vi "Near Field Motors.vi"() -> ()   [LabVIEW 2014]
doc: "Use this template to build a producer/consumer design pattern with events to produce queue items. Use this design pattern instead of the User Interface Event Handler pattern for user interfaces when you want to execute code asynchronously in response to an event without slowing the user interface responsiveness."
panel:
  out "File error out":errorcluster
  in  "RefLabels 4":string(combo) caption="M4"
  in  "RefLabels 3":string(combo) caption="M3"
  in  "RefLabels 2":string(combo) caption="M2"
  in  "All refs":dbl[][](array[numeric]) format="%.6f"
  in  "RefLabels 1":string(combo) caption="M1"
  in  "Referencing mode":T1(array[ring])=[enum."FRF (-> FNL)", enum."FRF (-> FNL)", enum."FRF (-> FNL)", enum."FRF (-> FNL)"]
  out "Host address":string
  out "Message":string
  out "Identification":string
  out "PI error out":errorcluster
  in  "Save References":bool
  in  "Set 4":bool caption="Set4"
  in  "Go 4":bool caption="Go4"
  in  "Set 3":bool caption="Set3"
  in  "Go 3":bool caption="Go3"
  in  "Set 2":bool caption="Set2"
  in  "Go 2":bool caption="Go2"
  in  "Go 1":bool caption="Go1"
  in  "Set 1":bool caption="Set1"
  in  "Ref Values":dbl[](array[numeric]) format="%.6f"
  in  "Max Pos":dbl[](array[numeric]) format="%.6f"
  in  "Min Pos":dbl[](array[numeric]) format="%.6f"
  in  "MOVE":bool
  in  "stop motors":bool
  out "Current position":dbl[](array[numeric]) format="%.6f"
  in  "Absolute \ntarget position":dbl[](array[numeric]) format="%.6f"
  in  "MV -":bool
  in  "Relative distance to mv":dbl format="%#_g mm"
  in  "Axis to move":T2(ring)
  in  "MV+":bool
  out "Init OK":bool
  in  "Axes to move":string[](array[string])
  out "+/- movement\nrange":dbl[](array[numeric]) format="%.6f"
  out "Referencing\nin progress":bool
  out "Conn. \nAxes":string[](array[string])
  in  "All Axes?":bool=TRUE
  in  "Stage selection":T3={"Force?"=FALSE, "Dialog?"=TRUE, "Stages"=[]}
  out "Position":dbl[](array[numeric]) format="%.6f"
  out "Referencing\nsuccessful?":bool[](array[boolean])
  in  "Reference Motors":bool
  in  "stop":bool
  # "M1: Horizontal NF"
  # "M2: Vertical NF"
  # "<unassigned>"
  # "<unassigned>"
  # "M1: Horizontal NF"
  # "M2: Vertical NF"
  # "<unassigned>"
  # "<unassigned>"
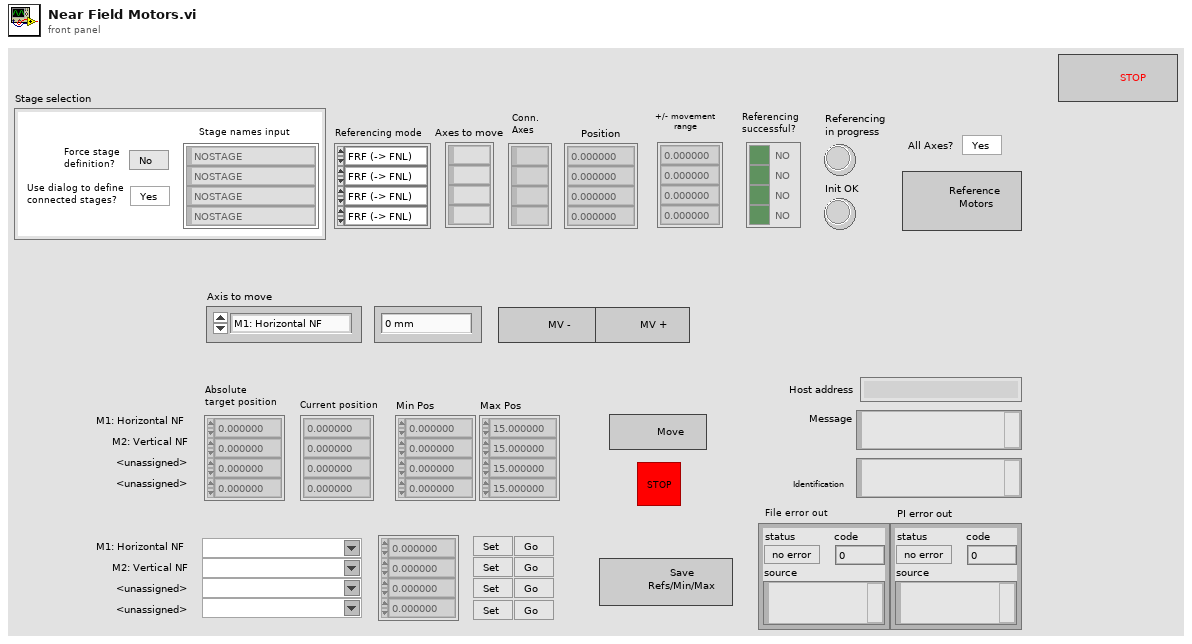
[diagram p1: front panel]
types:
  T1 = enum16{"FRF (-> FNL)", "FRF", "FNL", "FPL", "RON OFF"}[]
  T2 = enum16{"M1: Horizontal NF", "M2 : Vertical NF", "M3 : <unassigned> ", "M4 : <unassigned>"}
  T3 = cluster{"Force?":bool, "Dialog?":bool, "Stages":string[]}
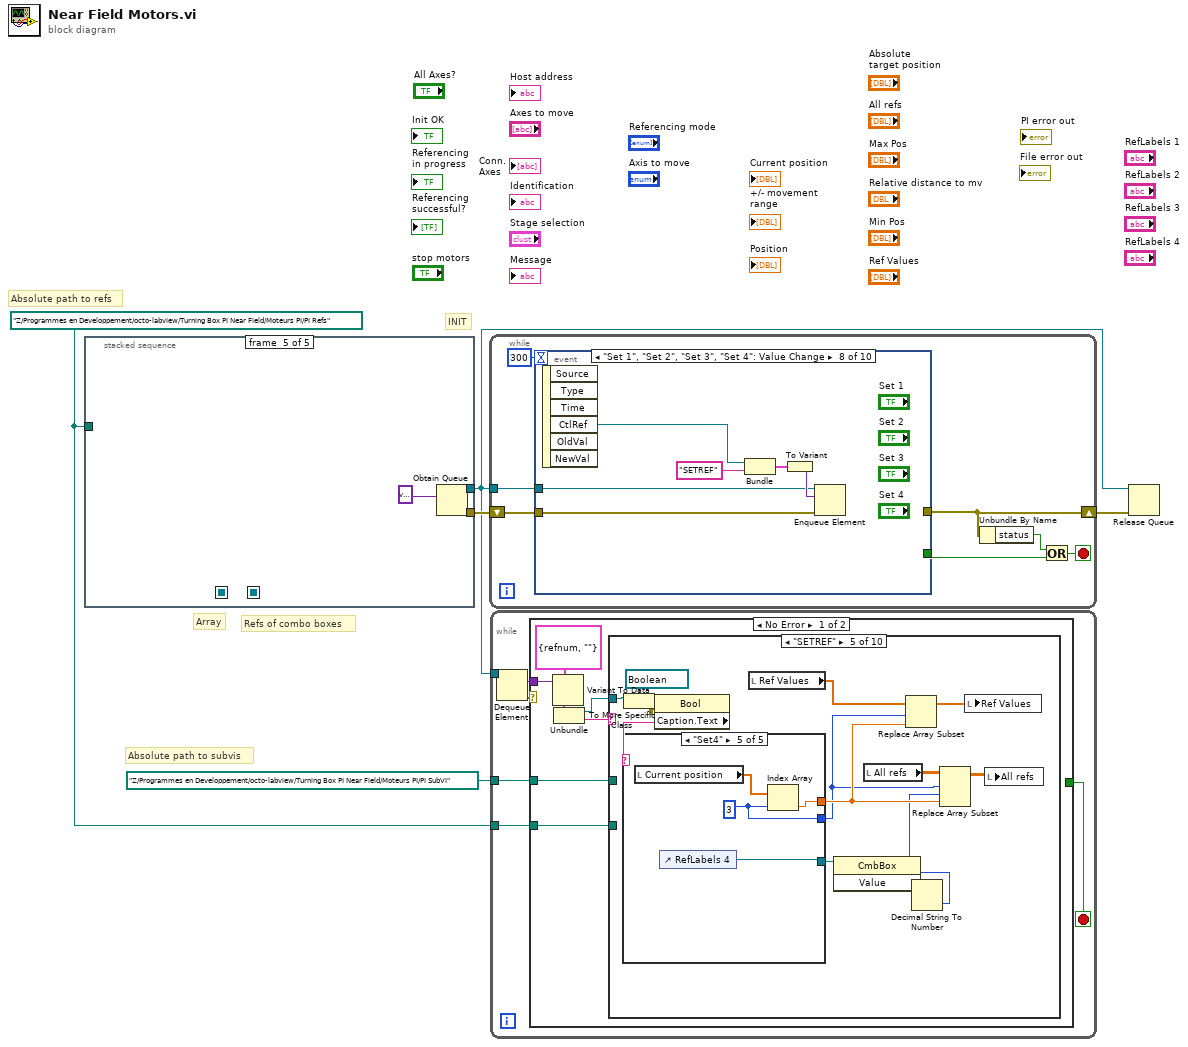
[diagram p0: block diagram]
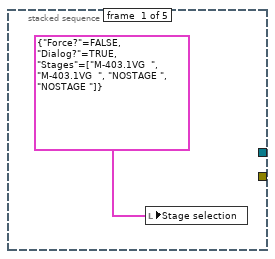
[diagram p2: hidden frame]
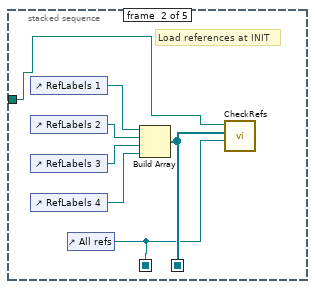
[diagram p3: hidden frame]
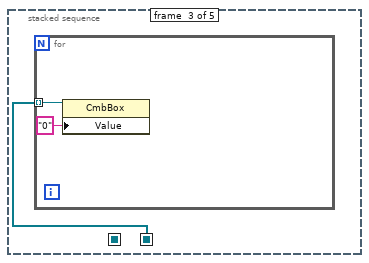
[diagram p4: hidden frame]
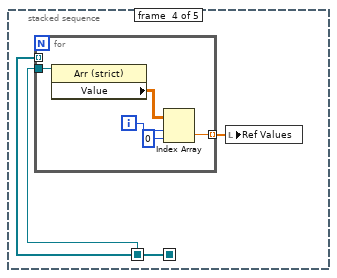
[diagram p5: hidden frame]
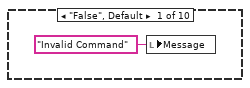
[diagram p6: hidden frame]
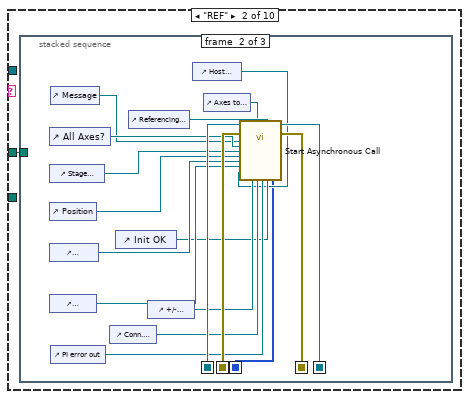
[diagram p7: hidden frame]
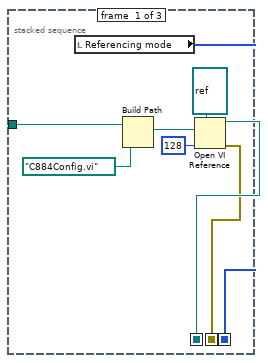
[diagram p8: hidden frame]
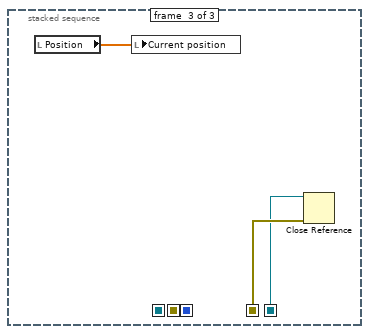
[diagram p9: hidden frame]
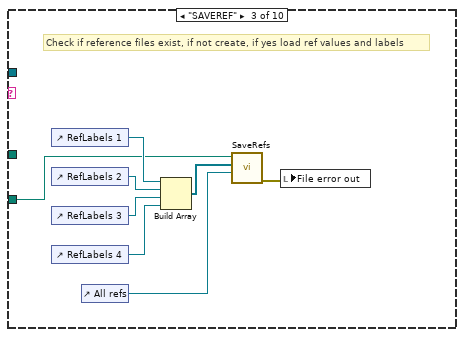
[diagram p10: hidden frame]
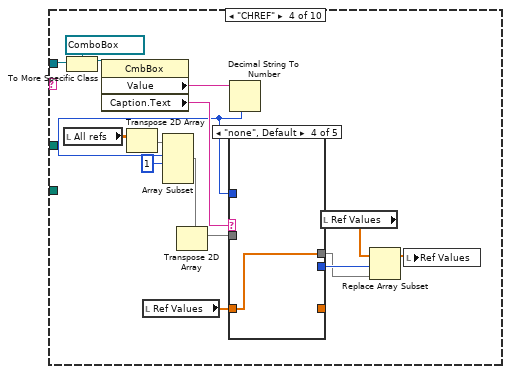
[diagram p11: hidden frame]
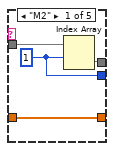
[diagram p12: hidden frame]
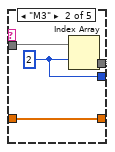
[diagram p13: hidden frame]
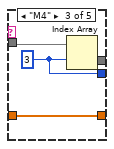
[diagram p14: hidden frame]
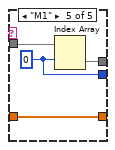
[diagram p15: hidden frame]
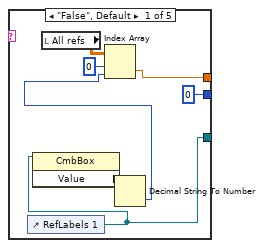
[diagram p16: hidden frame]
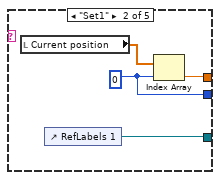
[diagram p17: hidden frame]
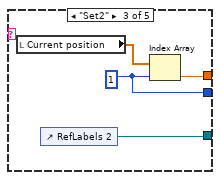
[diagram p18: hidden frame]
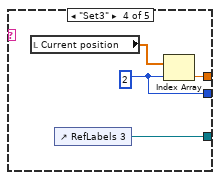
[diagram p19: hidden frame]
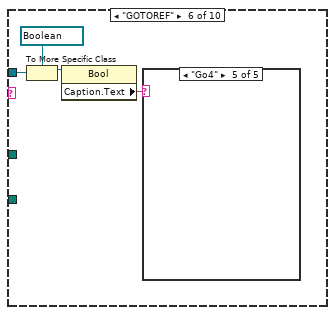
[diagram p20: hidden frame]
diagram:
  w1 = path "Z:/Programmes en Developpement/octo-labview/Turning Box PI Near Field/Moteurs PI/PI Refs" ("vi path")
  # "Refs of combo boxes"
  # "Array"
  # "Absolute path to refs"
  # "Absolute path to subvis"
  # "INIT"
  n1 = stacked-sequence {
    seq-local: [_ w8 _ _ _] -> [_ _ w14 w19 _]
    seq-local: [_ w7 _ _ _] -> [_ _ _ w18 _]
    tunnel: [_ _ _ _ w27] -> w5
    tunnel: [_ _ _ _ w26] -> w3
    tunnel: w1 -> [_ w9 _ _ _]
    frame #0 {
      n2 = local write "Stage selection"(T3 {"Force?"=FALSE, "Dialog?"=TRUE, "Stages"=["M-403.1VG  ", "M-403.1VG  ", "NOSTAGE ", "NOSTAGE "]} ("Stage selection")) -> ()
    }
    frame #1 {
      # "Load references at INIT"
      n3 = control-ref of="RefLabels 1"() -> (w10:refnum<vi>)
      n4 = control-ref of="RefLabels 2"() -> (w11:refnum<vi>)
      n5 = control-ref of="RefLabels 3"() -> (w12:refnum<vi>)
      n6 = control-ref of="RefLabels 4"() -> (w13:refnum<vi>)
      n7 = control-ref of="All refs"() -> (w7:refnum<vi>)
      n8 = Build Array(w10, w11, w12, w13) -> (w8:refnum<vi>[])
      n9 = call "CheckRefs.vi"("All Refs Array Refnum"=w7, "Array of label refnums"=w8, "Path to refs"=w9) -> ()  [unwired: 8 in, 1 out]
    }
    frame #2 {
      n10 = for {
        tunnel: w14 -> [w16] mode=indexing
        n11 = property class="CmbBox"(reference=w16, "Value"="0") -> ()  [unwired: 1 in, 2 out]
      }
    }
    frame #3 {
      n12 = for {
        tunnel: w19 -> [_] mode=indexing
        tunnel: w18 -> [w24]
        tunnel: [w20] -> w17 mode=indexing
        i -> [w22]
        n13 = property class="Arr (strict)"(reference=w24) -> ("Value"=w23:dbl[][])  [unwired: 1 in, 2 out]
        n14 = Index Array(array=w23, index (row)=w22, index (col)=0 ("disabled index (col)")) -> (element=w20:dbl)
      }
      n15 = local write "Ref Values"(w17) -> ()
    }
    frame #4 {
      n16 = Obtain Queue(element data type=variant) -> (queue out=w26:refnum<queue>, error out=w27:errorcluster)  [unwired: 4 in, 1 out]
    }
  }
  n17 = while {
    shift-right: [w30] -> w4
    shift-left: w5 -> [w33]
    tunnel: w3 -> [w34]
    stop <- w31 stop-if-true
    n18 = event shown="[7] \"Set 1\", \"Set 2\", \"Set 3\", \"Set 4\": Value Change" {
      selector: _ -> [_ _ _ _ _ _ _ _ _ _]
      dyn-events: _ -> [_ _ _ _ _ _ _ _ _ _]
      timeout: 300 -> [_ _ _ _ _ _ _ _ _ _]
      tunnel: w34 -> [w40 w46 w52 w58 w64 w69 w75 w78 w84 _]
      tunnel: w33 -> [w39 w45 w51 w57 w63 w70 w74 w77 w83 w89]
      tunnel: [_ _ _ _ _ _ _ _ _ w89] -> w30
      tunnel: [_ _ _ _ _ _ _ _ _ "stop"] -> w32
      event "Reference Motors": Value Change {
        n19 = event-data() -> ()  [unwired: 1 in, 1 out]
        n20 = Bundle("CtlRef"=refnum<vi> refnum, "element"="REF") -> (w36:cluster{"CtlRef":refnum<vi>, "element":string})  [unwired: 1 in]
        n21 = To Variant(anything=w36) -> (Variant=w38:variant)
        n22 = Enqueue Element(queue=w40, element=w38, error in (no error)=w39) -> ()  [unwired: 1 in, 3 out]
      }
      event Timeout {
        n23 = event-data() -> ()  [unwired: 1 in, 1 out]
        n24 = Bundle("CtlRef"=refnum<vi> refnum, "element"="POS?") -> (w42:cluster{"CtlRef":refnum<vi>, "element":string})  [unwired: 1 in]
        n25 = To Variant(anything=w42) -> (Variant=w44:variant)
        n26 = Enqueue Element(queue=w46, element=w44, error in (no error)=w45) -> ()  [unwired: 1 in, 3 out]
      }
      event "MV+": Value Change {
        n27 = event-data() -> ()  [unwired: 1 in, 1 out]
        n28 = Bundle("CtlRef"=refnum<vi> refnum, "element"="MVR +") -> (w48:cluster{"CtlRef":refnum<vi>, "element":string})  [unwired: 1 in]
        n29 = To Variant(anything=w48) -> (Variant=w50:variant)
        n30 = Enqueue Element(queue=w52, element=w50, error in (no error)=w51) -> ()  [unwired: 1 in, 3 out]
      }
      event "MV -": Value Change {
        n31 = event-data() -> ()  [unwired: 1 in, 2 out]
        n32 = Bundle("CtlRef"=refnum<vi> refnum, "element"="MVR -") -> (w54:cluster{"CtlRef":refnum<vi>, "element":string})  [unwired: 1 in]
        n33 = To Variant(anything=w54) -> (Variant=w56:variant)
        n34 = Enqueue Element(queue=w58, element=w56, error in (no error)=w57) -> ()  [unwired: 1 in, 3 out]
      }
      event "MOVE": Value Change {
        n35 = event-data() -> ()  [unwired: 1 in, 2 out]
        n36 = Bundle("CtlRef"=refnum<vi> refnum, "element"="MVABS") -> (w60:cluster{"CtlRef":refnum<vi>, "element":string})  [unwired: 1 in]
        n37 = To Variant(anything=w60) -> (Variant=w62:variant)
        n38 = Enqueue Element(queue=w64, element=w62, error in (no error)=w63) -> ()  [unwired: 1 in, 3 out]
      }
      event "Save References": Value Change {
        n39 = event-data() -> ()  [unwired: 1 in, 2 out]
        n40 = Bundle("CtlRef"=refnum<vi> refnum, "element"="SAVEREF") -> (w66:cluster{"CtlRef":refnum<vi>, "element":string})  [unwired: 1 in]
        n41 = To Variant(anything=w66) -> (Variant=w68:variant)
        n42 = Enqueue Element(queue=w69, element=w68, error in (no error)=w70) -> ()  [unwired: 1 in, 3 out]
      }
      event "RefLabels 1", "RefLabels 2", "RefLabels 3", "RefLabels 4": Value Change {
        n43 = event-data() -> ("CtlRef"=w71:refnum<vi>)  [unwired: 1 in, 5 out]
        n44 = Bundle("CtlRef"=w71, "element"="CHREF") -> (w73:cluster{"CtlRef":refnum<vi>, "element":string})  [unwired: 1 in]
        n45 = To Variant(anything=w73) -> (Variant=w72:variant)
        n46 = Enqueue Element(queue=w75, element=w72, error in (no error)=w74) -> ()  [unwired: 1 in, 3 out]
      }
      event "Set 1", "Set 2", "Set 3", "Set 4": Value Change {
        n47 = event-data() -> ("CtlRef"=w79:refnum<vi>)  [unwired: 1 in, 5 out]
        n48 = Bundle("CtlRef"=w79, "element"="SETREF") -> (w81:cluster{"CtlRef":refnum<vi>, "element":string})  [unwired: 1 in]
        n49 = To Variant(anything=w81) -> (Variant=w80:variant)
        n50 = Enqueue Element(queue=w78, element=w80, error in (no error)=w77) -> ()  [unwired: 1 in, 3 out]
      }
      event "Go 1", "Go 2", "Go 3", "Go 4": Value Change {
        n51 = event-data() -> ("CtlRef"=w85:refnum<vi>)  [unwired: 1 in, 5 out]
        n52 = Bundle("CtlRef"=w85, "element"="GOTOREF") -> (w87:cluster{"CtlRef":refnum<vi>, "element":string})  [unwired: 1 in]
        n53 = To Variant(anything=w87) -> (Variant=w86:variant)
        n54 = Enqueue Element(queue=w84, element=w86, error in (no error)=w83) -> ()  [unwired: 1 in, 3 out]
      }
      event "stop": Value Change {
        n55 = event-data() -> ()  [unwired: 1 in, 1 out]
      }
    }
    n56 = Unbundle By Name(w30) -> ("status"=w29:bool)
    n57 = Or(x=w29, y=w32) -> (x .or. y?=w31:bool)
  }
  n58 = while {
    tunnel: w3 -> [w96]
    tunnel: path "Z:/Programmes en Developpement/octo-labview/Turning Box PI Near Field/Moteurs PI/PI SubVI" ("vi path") -> [w92]
    tunnel: w1 -> [w91]
    stop <- w93 stop-if-true
    n59 = Dequeue Element(queue=w96) -> (element=w94:variant, error out=w95:errorcluster)  [unwired: 2 in, 2 out]
    n60 = case shown="No Error" w95 {
      tunnel: w94 -> [w101 _]
      tunnel: [_ TRUE] -> w93
      tunnel: w92 -> [w103 _]
      tunnel: w91 -> [w102 _]
      frame No Error {
        n61 = Variant To Data(type=cluster{"CtlRef":refnum<vi>, "element":string} {"CtlRef"=refnum, "element"=""} ("cluster"), Variant=w101) -> (data=w100:cluster{"CtlRef":refnum<vi>, "element":string})  [unwired: 1 in, 1 out]
        n62 = Unbundle(w100) -> ("CtlRef"=w98:refnum<vi>, "element"=w99:string)
        n63 = case shown="\"SETREF\"" w99 {
          tunnel: w103 -> [_ w105 _ _ _ _ w217 w239 w267 _]
          tunnel: w102 -> [_ _ w138 _ _ _ _ _ _ _]
          tunnel: w98 -> [_ _ _ w158 w189 w216 _ _ _ _]
          frame "False", Default {
            n64 = local write "Message"("Invalid Command" ("Message")) -> ()
          }
          frame "REF" {
            n65 = stacked-sequence {
              seq-local: [w111 _ _] -> [_ w131 _]
              seq-local: [w110 _ _] -> [_ w130 _]
              seq-local: [_ w117 _] -> [_ _ w134]
              seq-local: [_ w116 _] -> [_ _ w133]
              seq-local: [w106 _ _] -> [_ w114 _]
              tunnel: w105 -> [w109 _ _]
              frame #0 {
                n66 = local read "Referencing mode"() -> (w106:T1)
                n67 = Build Path(base path=w109, name or relative path=path "C884Config.vi" ("vi path")) -> (appended path=w107:path)
                n68 = Open VI Reference(type specifier VI Refnum (for type only)=refnum<vi> refnum, vi path=w107, options=128) -> (vi reference=w111:refnum<vi>, error out=w110:errorcluster)  [unwired: 3 in]
              }
              frame #1 {
                n69 = control-ref of="All Axes?"() -> (w129:refnum<vi>)
                n70 = control-ref of="Stage selection"() -> (w122:refnum<vi>)
                n71 = control-ref of="Position"() -> (w128:refnum<vi>)
                n72 = control-ref of="Identification"() -> (w127:refnum<vi>)
                n73 = control-ref of="Referencing\nsuccessful?"() -> (w126:refnum<vi>)
                n74 = control-ref of="Message"() -> (w119:refnum<vi>)
                n75 = control-ref of="PI error out"() -> (w123:refnum<vi>)
                n76 = control-ref of="Conn. \nAxes"() -> (w124:refnum<vi>)
                n77 = control-ref of="Init OK"() -> (w118:refnum<vi>)
                n78 = control-ref of="Referencing\nin progress"() -> (w121:refnum<vi>)
                n79 = control-ref of="+/- movement\nrange"() -> (w125:refnum<vi>)
                n80 = control-ref of="Host address"() -> (w115:refnum<vi>)
                n81 = control-ref of="Axes to move"() -> (w120:refnum<vi>)
                n82 = call-by-ref "Start Asynchronous Call"(reference=w131, error in=w130, "All axes? Refnum"=w129, "Stages Selection Refnum"=w122, "Position Refnum"=w128, "Identification Refnum"=w127, "Referencing successful Refnum"=w126, "Host Addresss Refnum"=w115, "Message Out Refnum"=w119, "+/- mvt range Refnum"=w125, "Axes to Move Refnum"=w120, "Connected Axes Refnum"=w124, "Referencing mode"=w114, "Error OUT Refnum"=w123, "En cours LED Refnum"=w121, "LED Initialis. OK? Refnum"=w118) -> (reference out=w116:refnum<vi>, error out=w117:errorcluster)  [unwired: 6 in]
              }
              frame #2 {
                n83 = local read "Position"() -> (w132:dbl[])
                n84 = local write "Current position"(w132) -> ()
                n85 = Close Reference(reference=w133, error in (no error)=w134) -> ()  [unwired: 1 out]
              }
            }
          }
          frame "SAVEREF" {
            # "Check if reference files exist, if not create, if yes load ref values and labels"
            n86 = control-ref of="RefLabels 1"() -> (w142:refnum<vi>)
            n87 = control-ref of="RefLabels 2"() -> (w141:refnum<vi>)
            n88 = control-ref of="RefLabels 3"() -> (w140:refnum<vi>)
            n89 = control-ref of="RefLabels 4"() -> (w139:refnum<vi>)
            n90 = control-ref of="All refs"() -> (w136:refnum<vi>)
            n91 = Build Array(w142, w141, w140, w139) -> (w137:refnum<vi>[])
            n92 = call "SaveRefs.vi"("All Refs Array Refnum"=w136, "Array of label refnums"=w137, "Path to refs"=w138) -> ("error out"=w135:errorcluster)  [unwired: 8 in]
            n93 = local write "File error out"(w135) -> ()
          }
          frame "CHREF" {
            n94 = local read "All refs"() -> (w153:dbl[][])
            n95 = To More Specific Class(target class=refnum<vi> refnum ("CtlRef"), reference=w158) -> (specific class reference=w156:refnum<vi>)  [unwired: 1 in, 1 out]
            n96 = property class="CmbBox"(reference=w156) -> ("Value"=w155:string, "Caption.Text"=w154:string)  [unwired: 1 in, 2 out]
            n97 = Transpose 2D Array(2D array=w153) -> (transposed array=w152:dbl[][])
            n98 = local read "Ref Values"() -> (w147:dbl[])
            n99 = Decimal String To Number(string=w155) -> (number=w151:i32)  [unwired: 2 in, 1 out]
            n100 = Array Subset(array=w152, index (row)=w151, length (row)=1 ("length")) -> (w149:dbl[][])  [unwired: 2 in]
            n101 = Transpose 2D Array(2D array=w149) -> (transposed array=w148:dbl[][])
            n102 = case shown="\"none\", Default" w154 {
              tunnel: w151 -> [_ _ _ _ _]
              tunnel: w148 -> [w162 w166 w170 _ w175]
              tunnel: [w161 w164 w168 _ w174] -> w145
              tunnel: [w160 w165 w169 w171 w173] -> w144
              tunnel: w147 -> [w159 w163 w167 w171 w172]
              tunnel: [w159 w163 w167 _ w172] -> _
              frame "M2" {
                w161 = 1
                n103 = Index Array(array=w162, index (row)=w161) -> (element=w160:dbl[])  [unwired: 1 in]
              }
              frame "M3" {
                w164 = 2
                n104 = Index Array(array=w166, index (row)=w164) -> (element=w165:dbl[])  [unwired: 1 in]
              }
              frame "M4" {
                w168 = 3
                n105 = Index Array(array=w170, index (row)=w168) -> (element=w169:dbl[])  [unwired: 1 in]
              }
              frame "none", Default {
              }
              frame "M1" {
                w174 = 0
                n106 = Index Array(array=w175, index (row)=w174) -> (element=w173:dbl[])  [unwired: 1 in]
              }
            }
            n107 = local read "Ref Values"() -> (w146:dbl[])
            n108 = Replace Array Subset(array=w146, new element=w144, index=w145) -> (w143:dbl[])
            n109 = local write "Ref Values"(w143) -> ()
          }
          frame "SETREF" {
            n110 = To More Specific Class(target class=refnum<vi> refnum ("CtlRef"), reference=w189) -> (specific class reference=w187:refnum<vi>, error out=w186:errorcluster)  [unwired: 1 in]
            n111 = property class="Bool"(reference=w187, error in=w186) -> ("Caption.Text"=w185:string)  [unwired: 2 out]
            n112 = case shown="\"Set4\"" w185 {
              tunnel: [w191 w199 w203 w207 w211] -> w178
              tunnel: [0 w198 w202 w206 w210] -> w176
              tunnel: [w190 w197 w201 w205 w209] -> w179
              frame "False", Default {
                n113 = control-ref of="RefLabels 1"() -> (w190:refnum<vi>)
                n114 = property class="CmbBox"(reference=w190) -> ("Value"=w195:string)  [unwired: 1 in, 2 out]
                n115 = local read "All refs"() -> (w196:dbl[][])
                n116 = Decimal String To Number(string=w195) -> (number=w192:i32)  [unwired: 2 in, 1 out]
                n117 = Index Array(array=w196, index (row)=0, index (col)=w192) -> (element=w191:dbl)
              }
              frame "Set1" {
                w198 = 0
                n118 = local read "Current position"() -> (w200:dbl[])
                n119 = control-ref of="RefLabels 1"() -> (w197:refnum<vi>)
                n120 = Index Array(array=w200, index=w198) -> (element=w199:dbl)
              }
              frame "Set2" {
                w202 = 1
                n121 = local read "Current position"() -> (w204:dbl[])
                n122 = control-ref of="RefLabels 2"() -> (w201:refnum<vi>)
                n123 = Index Array(array=w204, index=w202) -> (element=w203:dbl)
              }
              frame "Set3" {
                w206 = 2
                n124 = local read "Current position"() -> (w208:dbl[])
                n125 = control-ref of="RefLabels 3"() -> (w205:refnum<vi>)
                n126 = Index Array(array=w208, index=w206) -> (element=w207:dbl)
              }
              frame "Set4" {
                w210 = 3
                n127 = local read "Current position"() -> (w212:dbl[])
                n128 = control-ref of="RefLabels 4"() -> (w209:refnum<vi>)
                n129 = Index Array(array=w212, index=w210) -> (element=w211:dbl)
              }
            }
            n130 = local read "Ref Values"() -> (w183:dbl[])
            n131 = property class="CmbBox"(reference=w179) -> ("Value"=w184:string)  [unwired: 1 in, 2 out]
            n132 = local read "All refs"() -> (w182:dbl[][])
            n133 = Replace Array Subset(array=w183, new element=w178, index=w176) -> (w180:dbl[])
            n134 = Decimal String To Number(string=w184) -> (number=w177:i32)  [unwired: 2 in, 1 out]
            n135 = Replace Array Subset(array=w182, new element=w178, index (row)=w176, index (col)=w177) -> (w181:dbl[][])
            n136 = local write "Ref Values"(w180) -> ()
            n137 = local write "All refs"(w181) -> ()
          }
          frame "GOTOREF" {
            n138 = To More Specific Class(target class=refnum<vi> refnum ("CtlRef"), reference=w216) -> (specific class reference=w214:refnum<vi>)  [unwired: 1 in, 1 out]
            n139 = property class="Bool"(reference=w214) -> ("Caption.Text"=w213:string)  [unwired: 1 in, 2 out]
            n140 = case shown="\"Go4\"" w213 {
              frame "False", Default {
              }
              frame "Go1" {
              }
              frame "Go2" {
              }
              frame "Go3" {
              }
              frame "Go4" {
              }
            }
          }
          frame "MVABS" {
            n141 = stacked-sequence {
              seq-local: [w220 _ _] -> [_ w236 _]
              seq-local: [w219 _ _] -> [_ w235 _]
              seq-local: [_ w227 _] -> [_ _ w238]
              seq-local: [_ w226 _] -> [_ _ w237]
              seq-local: [w218 _ _] -> [_ w225 _]
              tunnel: w217 -> [w222 _ _]
              frame #0 {
                n142 = local read "Absolute \ntarget position"() -> (w218:dbl[])
                n143 = Build Path(base path=w222, name or relative path=path "MoveSinglePIMotor_C884.vi" ("vi path")) -> (appended path=w221:path)
                n144 = Open VI Reference(type specifier VI Refnum (for type only)=refnum<vi> refnum, vi path=w221) -> (vi reference=w220:refnum<vi>, error out=w219:errorcluster)  [unwired: 4 in]
              }
              frame #1 {
                n145 = control-ref of="stop motors"() -> (w228:refnum<vi>)
                n146 = call-by-ref "Start Asynchronous Call"(reference=w236, error in=w235, "System no."=1, "Move"=w225, "Define home"=FALSE, "Move relative (-)"=FALSE, "Go home"=FALSE, "Move relative (+)"=FALSE ("Move relative (-)"), "Move absolute"=TRUE ("Move relative (-)"), "Stop refnum"=w228) -> (reference out=w227:refnum<vi>, error out=w226:errorcluster)  [unwired: 10 in, 2 out]
              }
              frame #2 {
                n147 = Close Reference(reference=w238, error in (no error)=w237) -> ()  [unwired: 1 out]
              }
            }
          }
          frame "MVR +" {
            n148 = stacked-sequence {
              seq-local: [w247 _ _] -> [_ w264 _]
              seq-local: [w246 _ _] -> [_ w263 _]
              seq-local: [_ w255 _] -> [_ _ w266]
              seq-local: [_ w254 _] -> [_ _ w265]
              seq-local: [w244 _ _] -> [_ w252 _]
              seq-local: [w240 _ _] -> [_ w253 _]
              tunnel: w239 -> [w249 _ _]
              frame #0 {
                n149 = local read "Axis to move"() -> (w242:T2)
                n150 = local read "Relative distance to mv"() -> (w245:dbl)
                n151 = local read "Conn. \nAxes"() -> (w243:string[])
                n152 = Index Array(array=w243, index=w242) -> (element=w241:string)
                n153 = Build Path(base path=w249, name or relative path=path "MoveSinglePIMotor_C884.vi" ("vi path")) -> (appended path=w248:path)
                n154 = Build Array(w245) -> (w244:dbl[])
                n155 = Build Array(w241) -> (w240:string[])
                n156 = Open VI Reference(type specifier VI Refnum (for type only)=refnum<vi> refnum, vi path=w248) -> (vi reference=w247:refnum<vi>, error out=w246:errorcluster)  [unwired: 4 in]
              }
              frame #1 {
                n157 = control-ref of="stop motors"() -> (w256:refnum<vi>)
                n158 = call-by-ref "Start Asynchronous Call"(reference=w264, error in=w263, "System no."=1, "Axes to move"=w253, "Move"=w252, "Define home"=FALSE, "Move relative (-)"=FALSE, "Go home"=FALSE, "Move relative (+)"=TRUE ("Move relative (-)"), "Move absolute"=FALSE ("Move relative (-)"), "Stop refnum"=w256) -> (reference out=w255:refnum<vi>, error out=w254:errorcluster)  [unwired: 9 in, 2 out]
              }
              frame #2 {
                n159 = Close Reference(reference=w266, error in (no error)=w265) -> ()  [unwired: 1 out]
              }
            }
          }
          frame "MVR -" {
            n160 = stacked-sequence {
              seq-local: [w275 _ _] -> [_ w292 _]
              seq-local: [w274 _ _] -> [_ w291 _]
              seq-local: [_ w283 _] -> [_ _ w294]
              seq-local: [_ w282 _] -> [_ _ w293]
              seq-local: [w272 _ _] -> [_ w280 _]
              seq-local: [w268 _ _] -> [_ w281 _]
              tunnel: w267 -> [w277 _ _]
              frame #0 {
                n161 = local read "Axis to move"() -> (w270:T2)
                n162 = local read "Conn. \nAxes"() -> (w271:string[])
                n163 = local read "Relative distance to mv"() -> (w273:dbl)
                n164 = Index Array(array=w271, index=w270) -> (element=w269:string)
                n165 = Build Path(base path=w277, name or relative path=path "MoveSinglePIMotor_C884.vi" ("vi path")) -> (appended path=w276:path)
                n166 = Build Array(w269) -> (w268:string[])
                n167 = Build Array(w273) -> (w272:dbl[])
                n168 = Open VI Reference(type specifier VI Refnum (for type only)=refnum<vi> refnum, vi path=w276) -> (vi reference=w275:refnum<vi>, error out=w274:errorcluster)  [unwired: 4 in]
              }
              frame #1 {
                n169 = control-ref of="stop motors"() -> (w284:refnum<vi>)
                n170 = call-by-ref "Start Asynchronous Call"(reference=w292, error in=w291, "System no."=1, "Axes to move"=w281, "Move"=w280, "Define home"=FALSE, "Move relative (-)"=TRUE, "Go home"=FALSE, "Move relative (+)"=FALSE ("Move relative (-)"), "Move absolute"=FALSE ("Move relative (-)"), "Stop refnum"=w284) -> (reference out=w283:refnum<vi>, error out=w282:errorcluster)  [unwired: 9 in, 2 out]
              }
              frame #2 {
                n171 = Close Reference(reference=w294, error in (no error)=w293) -> ()  [unwired: 1 out]
              }
            }
          }
          frame "POS?" {
            n172 = call "POS?.vi"("System no."=1, "All axes?"=TRUE) -> ("Position"=w295:dbl[])  [unwired: 16 in, 1 out]
            n173 = local write "Absolute \ntarget position"(w295) -> ()
            n174 = local write "Current position"(w295) -> ()
            n175 = local write "Position"(w295) -> ()
          }
        }
      }
      frame Error {
        # "Return true in any case that should stop the loop."
      }
    }
  }
  n176 = Release Queue(queue=w3, error in (no error)=w4) -> ()  [unwired: 1 in, 3 out]
